vi "set_PID.vi"(8 "error in (no error)":errorcluster, 10 "PID cluster":cluster{"P":dbl, "I":dbl, "D":dbl}, 11 "VISA Refnum in":refnum<visa-resource-name>) -> (0 "error out":errorcluster, 3 "VISA Refnum out":refnum<visa-resource-name>)   [LabVIEW 2018]
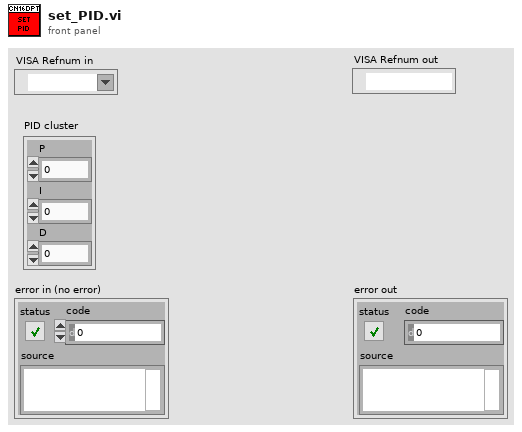
[diagram p1: front panel]
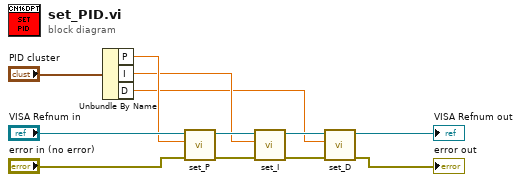
[diagram p0: block diagram]
diagram:
  n1 = Unbundle By Name("PID cluster") -> ("P"=w3:dbl, "I"=w2:dbl, "D"=w1:dbl)
  n2 = call "set_P.vi"("error in (no error)"="error in (no error)", "P"=w3, "VISA Refnum in"="VISA Refnum in") -> ("error out"=w7:errorcluster, "VISA Refnum out"=w10:refnum<visa-resource-name>)  [unwired: 7 in]
  n3 = call "set_I.vi"("error in (no error)"=w7, "I"=w2, "VISA Refnum in"=w10) -> ("error out"=w6:errorcluster, "VISA Refnum out"=w9:refnum<visa-resource-name>)  [unwired: 7 in]
  n4 = call "set_D.vi"("error in (no error)"=w6, "D"=w1, "VISA Refnum in"=w9) -> ("error out"=→"error out":errorcluster, "VISA Refnum out"=→"VISA Refnum out":refnum<visa-resource-name>)  [unwired: 7 in]
